vi "GetDefaultParams.vi"(8 "error in (no error)":errorcluster, 10 "Path":path, 11 "NiPxi6733 in":refnum<class "NiPxi6733.lvclass">) -> (0 "error out":errorcluster, 3 "NiPxi6733 out":refnum<class "NiPxi6733.lvclass">)   [LabVIEW 2014, in "FgenPlugins.lvlib" / "NiPxi6733.lvclass"]
uses:
  NiPxi6733.lvclass
  Typedefs/Timebase.ctl
  <userlib>/NIST/BaseClasses/BasePlugin_class/BasePlugin.lvclass/BasePlugin.ctl
  NiPxi6733.lvclass/NiPxi6733.ctl
  <userlib>/NIST/BaseClasses/BasePlugin_class/Accessors/Read PluginIniFilePath.vi
  Accessors/Write SampleRate.vi
  Accessors/Write Timebase.vi
  FgenPluginBaseClass/FgenPluginsBase.lvclass
  <vilib>/Utility/config.llb/NI_LVConfig.lvlib
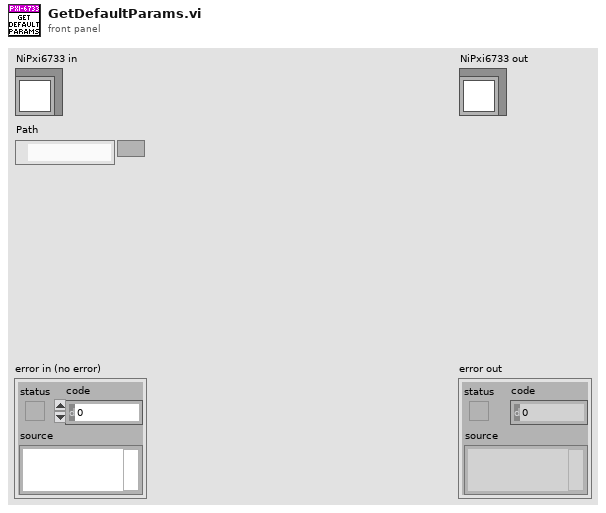
[diagram p1: front panel]
types:
  T1 = typedef "FgenPlugins.lvlib/NiPxi6733.lvclass/Timebase.ctl" = cluster{"source":string, "rate":dbl}
  T2 = typedef "NI_LVConfig.lvlib/Config Data RefNum.ctl" = refnum<k1>
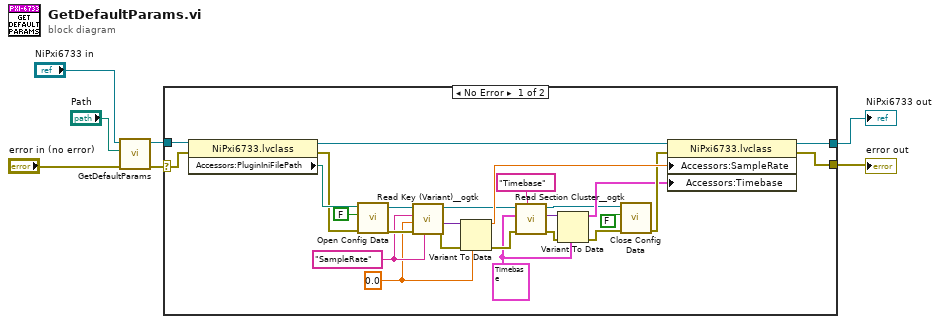
[diagram p0: block diagram]
diagram:
  n1 = call-parent "GetDefaultParams.vi"("error in (no error)"="error in (no error)", "Path"="Path", "FgenPluginsBase in"="NiPxi6733 in") -> ("error out"=w4:errorcluster, "FgenPluginsBase out"=w3:refnum<class "NiPxi6733.lvclass">)  [unwired: 7 in]
  n2 = case shown="No Error" w4 {
    selector: w4 -> [w32 w34]
    tunnel: w3 -> [w33 w35]
    tunnel: [w18 w35] -> w2
    tunnel: [w17 w34] -> w1
    frame No Error {
      w12 = T1 {"source"="/PXI1Slot6/PXI_Trig1", "rate"=18000000.0} ("Timebase")
      w22 = 0.0 ("SampleRate")
      w25 = "SampleRate" ("section")
      n3 = property class="NiPxi6733.lvclass"(reference=w33, error in=w32) -> (reference out=w26:refnum<class "NiPxi6733.lvclass">, error out=w30:errorcluster, "Accessors:PluginIniFilePath"=w31:path)
      n4 = call <vilib>:"Open Config Data.vi"("error in (no error)"=w30, "create file if necessary (T)"=FALSE, "configuration file path"=w31) -> ("error out"=w28:errorcluster, "refnum"=w27:T2)  [unwired: 6 in, 1 out]
      n5 = call <userlib>:"Read Key (Variant)__ogtk.vi"("section"=w25, "error in (no error)"=w28, "type"=w22, "key (optional)"=w25, "refnum"=w27) -> ("error out"=w24:errorcluster, "key-value"=w23:variant, "refnum out"=w16:T2)  [unwired: 3 in, 1 out]
      n6 = Variant To Data(error in=w24, type=w22, Variant=w23) -> (data=w21:dbl, error out=w15:errorcluster)
      n7 = call <userlib>:"Read Section Cluster__ogtk.vi"("section (optional)"="Timebase", "error in (no error)"=w15, "Section Formatted Cluster Type"=w12, "refnum"=w16) -> ("error out"=w11:errorcluster, "Section Formatted Cluster"=w13:variant, "dup refnum"=w8:T2)  [unwired: 3 in, 2 out]
      n8 = Variant To Data(error in=w11, type=w12, Variant=w13) -> (data=w9:T1, error out=w10:errorcluster)
      n9 = call <vilib>:"Close Config Data.vi"("error in (no error)"=w10, "write file if changed (T)"=FALSE, "refnum"=w8) -> ("error out"=w19:errorcluster)  [unwired: 7 in, 1 out]
      n10 = property class="NiPxi6733.lvclass"(reference=w26, error in=w19, "Accessors:SampleRate"=w21, "Accessors:Timebase"=w9) -> (reference out=w18:refnum<class "NiPxi6733.lvclass">, error out=w17:errorcluster)
    }
    frame Error {
    }
  }
  "error out" <- w1
  "NiPxi6733 out" <- w2
